vi "Player Info.vi"(11 "Great Wall in":refnum<class "Great Wall.lvclass">) -> (0 "Defeat Speech":string, 1 "Victory Speech":string, 2 "Name":string, 3 "Great Wall out":refnum<class "Great Wall.lvclass">)   [LabVIEW 2015, in "Great Wall.lvclass"]
uses:
  Great Wall.lvclass
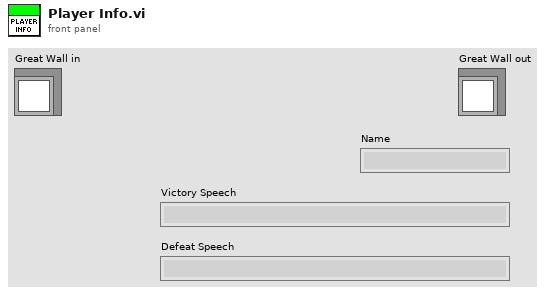
[diagram p1: front panel]
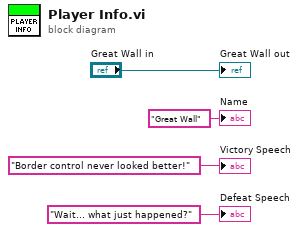
[diagram p0: block diagram]
diagram:
  "Great Wall out" <- "Great Wall in"
  "Name" <- "Great Wall" ("Name")
  "Victory Speech" <- "Border control never looked better!" ("Name")
  "Defeat Speech" <- "Wait... what just happened?" ("Name")
